vi "Assign two values from string to axes.vi"(2 "Queried axes":string[](array[string]), 4 "Input String":string, 5 "error in":errorcluster) -> (14 "Values 1":dbl[](array[numeric]) format="%.6f", 15 "Strings 1":string[](array[string]), 16 "Values 2":dbl[](array[numeric]) format="%.6f", 17 "Strings 2":string[](array[string]), 18 "Queried axes out":string[](array[string]), 19 "error out":errorcluster)   [LabVIEW 2020]
doc: "This VI assigns two values and/or strings from input string to queried axes."
panel:
  # "This vi assigns two values and/or strings from input string to queried axes."
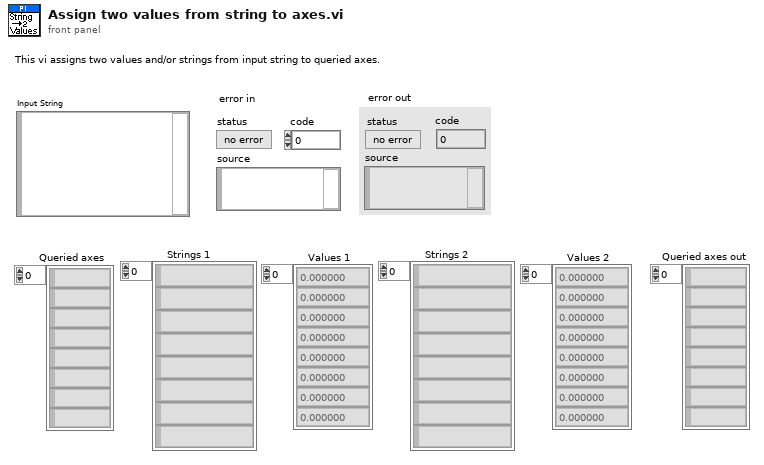
[diagram p1: front panel]
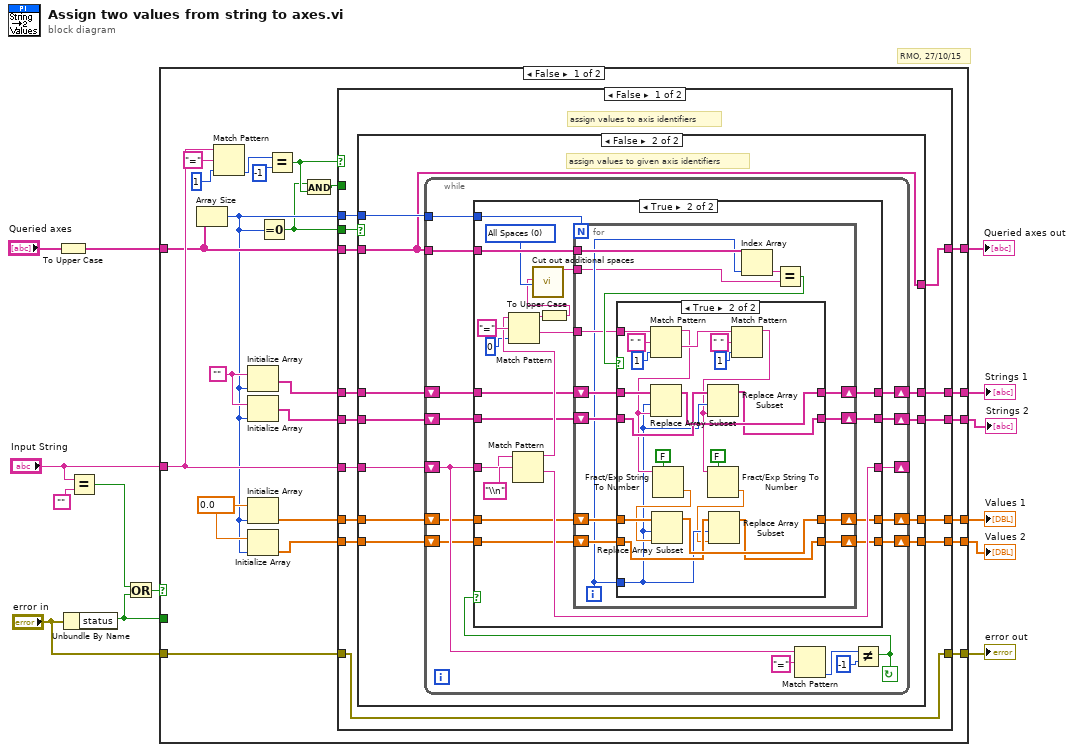
[diagram p0: block diagram]
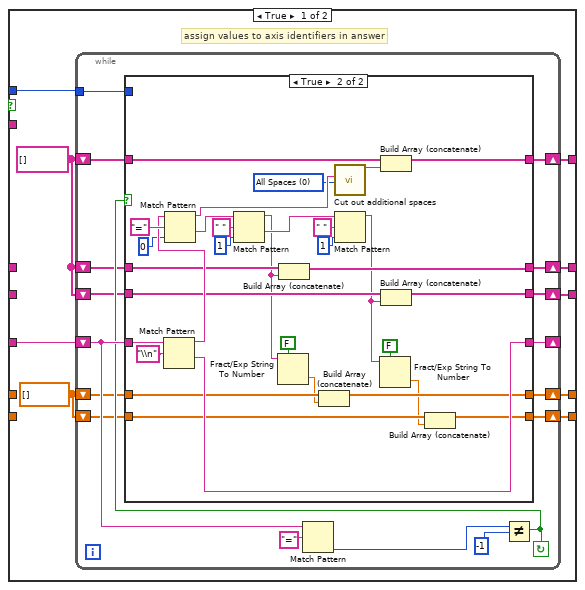
[diagram p2: hidden frame]
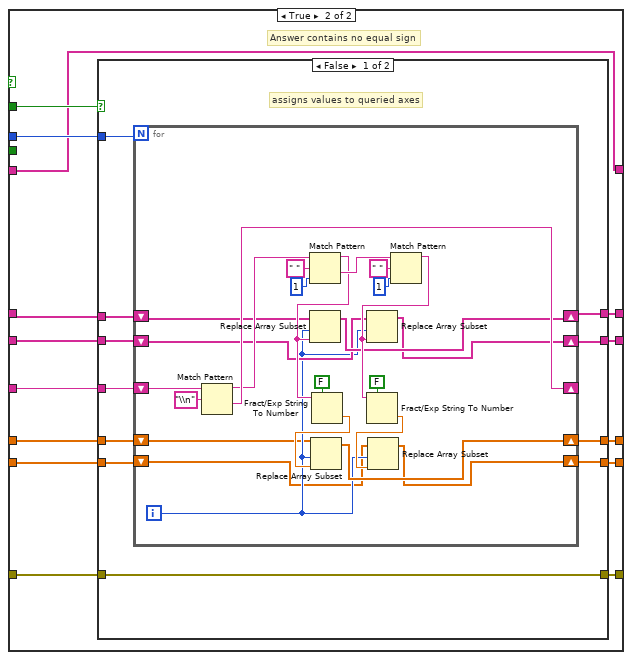
[diagram p6: hidden frame]
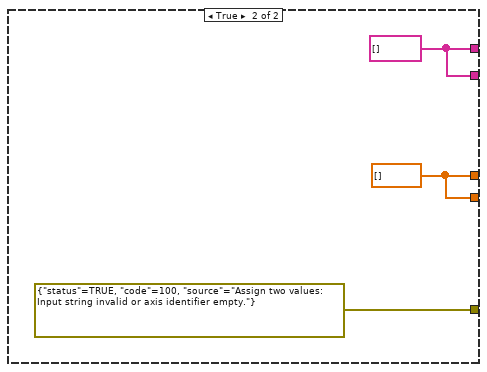
[diagram p7: hidden frame]
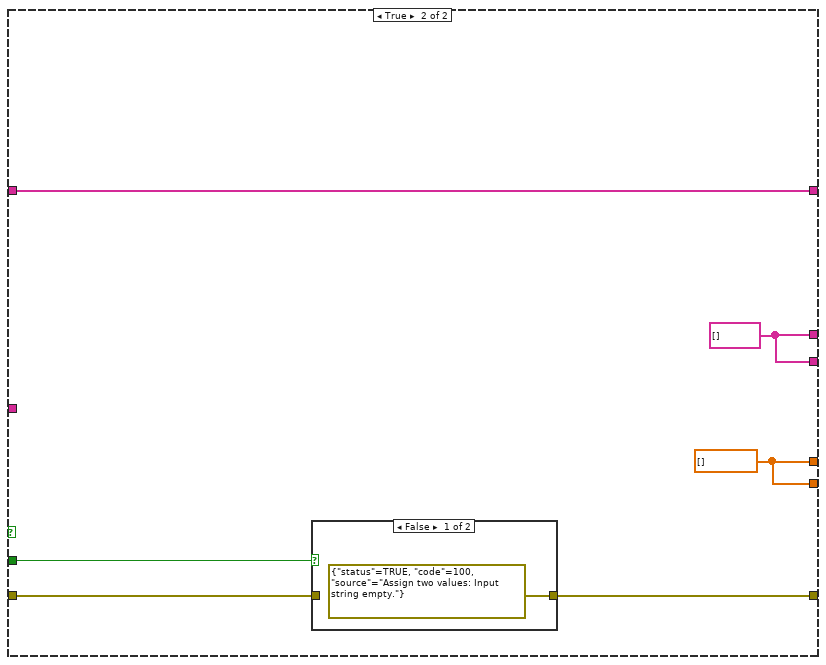
[diagram p8: hidden frame]
diagram:
  # "RMO, 27/10/15"
  n1 = To Upper Case(1:"Queried axes") -> (0:w5:string[])
  n2 = Unbundle By Name("error in") -> ("status"=w7:bool)
  n3 = Equal?(x="Input String", y="") -> (x = y?=w4:bool)
  n4 = Or(x=w4, y=w7) -> (x .or. y?=w9:bool)
  n5 = case shown="False" w9 {
    tunnel: "Input String" -> [w37 _]
    tunnel: [w36 w260] -> w14
    tunnel: w5 -> [w27 w259]
    tunnel: [w25 w263] -> w11
    tunnel: "error in" -> [w24 w264]
    tunnel: [w35 w261] -> w8
    tunnel: w7 -> [_ w262]
    tunnel: [w19 w261] -> w3
    tunnel: [w18 w260] -> w2
    tunnel: [w17 w259] -> w1
    frame False {
      w21 = 0.0 ("Element Data")
      w23 = ""
      n6 = Array Size(array=w27) -> (size(s)=w16:i32)
      n7 = Match Pattern(string=w37, regular expression="=", offset (0)=1) -> (offset past match=w32:i32)  [unwired: 3 out]
      n8 = Initialize Array(w23, w16) -> (w30:string[])
      n9 = Initialize Array(w23, w16) -> (w22:string[])
      n10 = Initialize Array(w21, w16) -> (w31:dbl[])
      n11 = Initialize Array(w21, w16) -> (w20:dbl[])
      n12 = Equal To 0?(x=w16) -> (x = 0?=w15:bool)
      n13 = Equal?(x=w32, y=-1) -> (x = y?=w28:bool)
      n14 = And(x=w15, y=w28) -> (x .and. y?=w26:bool)
      n15 = case shown="False" w28 {
        tunnel: [w50 w220] -> w36
        tunnel: w37 -> [w51 w219]
        tunnel: w27 -> [w40 w209]
        tunnel: w31 -> [w48 w218]
        tunnel: w16 -> [w49 w217]
        tunnel: w30 -> [w47 w216]
        tunnel: [w46 w215] -> w35
        tunnel: w26 -> [_ w214]
        tunnel: [w45 w213] -> w25
        tunnel: w24 -> [w45 w212]
        tunnel: [w44 w211] -> w19
        tunnel: w22 -> [w43 w208]
        tunnel: w20 -> [w42 w207]
        tunnel: [w41 w210] -> w18
        tunnel: [w38 w209] -> w17
        tunnel: w15 -> [w39 _]
        frame False {
          # "assign values to axis identifiers"
          n16 = case shown="False" w39 {
            tunnel: w51 -> [w60 w125]
            tunnel: [w59 w124] -> w50
            tunnel: w49 -> [w58 w123]
            tunnel: w48 -> [_ w122]
            tunnel: w47 -> [_ w121]
            tunnel: [w57 w120] -> w46
            tunnel: [w56 w119] -> w44
            tunnel: w43 -> [_ w118]
            tunnel: w42 -> [_ w117]
            tunnel: [w55 w116] -> w41
            tunnel: w40 -> [_ w115]
            tunnel: [w54 w115] -> w38
            frame True {
              w52 = dbl[] []
              w53 = string[] []
              # "assign values to axis identifiers in answer"
              n17 = while {
                shift-left: w53 -> [w67]
                shift-right: [w68] -> w57
                tunnel: w58 -> [w69]
                shift-left: w52 -> [w71]
                shift-right: [w70] -> w59
                shift-left: w60 -> [w74]
                shift-right: [w73] -> _
                shift-right: [w66] -> w56
                shift-left: w53 -> [w65]
                shift-right: [w64] -> w55
                shift-left: w52 -> [w63]
                shift-right: [w62] -> w54
                shift-left: w53 -> [w61]
                stop <- w72 continue-if-true
                n18 = Match Pattern(string=w74, regular expression="=") -> (offset past match=w75:i32)  [unwired: 4 out]
                n19 = Not Equal?(x=w75, y=-1) -> (x != y?=w72:bool)
                n20 = case shown="True" w72 {
                  tunnel: w74 -> [w83 w113]
                  tunnel: [w83 w112] -> w73
                  tunnel: [w82 w88] -> w70
                  tunnel: w71 -> [w82 w89]
                  tunnel: w69 -> [_ _]
                  tunnel: [w81 w94] -> w68
                  tunnel: w67 -> [w81 w95]
                  tunnel: [w80 w92] -> w66
                  tunnel: w65 -> [w80 w93]
                  tunnel: [w79 w84] -> w64
                  tunnel: w63 -> [w79 w86]
                  tunnel: [w78 w106] -> w62
                  tunnel: w61 -> [w78 w96]
                  frame False {
                    # "line contains no equal sign"
                  }
                  frame True {
                    w98 = u16 0 items=["All Spaces", "Only if 1st char.", "Only if last char.", "Only if near \"=\"", "Only if 1st or last char.", "Only multiple"] ("Mode")
                    n21 = Match Pattern(string=w113, regular expression="\\n") -> (before substring=w110:string, after substring=w112:string)  [unwired: 3 out]
                    n22 = Match Pattern(string=w110, regular expression="=", offset (0)=0) -> (before substring=w107:string, after substring=w109:string)  [unwired: 2 out]
                    n23 = Match Pattern(string=w109, regular expression=" ", offset (0)=1) -> (before substring=w91:string, after substring=w101:string)  [unwired: 2 out]
                    n24 = Fract/Exp String To Number(use system decimal point (T)=FALSE, string=w91) -> (number=w87:dbl)  [unwired: 3 out]
                    n25 = Build Array (concatenate)(w95, w91) -> (w94:string[])
                    n26 = Build Array (concatenate)(w89, w87) -> (w88:dbl[])
                    n27 = call "Cut out additional spaces.vi"("String"=w107, "Mode"=w98) -> ("String out"=w97:string)  [unwired: 17 out]
                    n28 = Match Pattern(string=w101, regular expression=" ", offset (0)=1) -> (before substring=w90:string)  [unwired: 3 out]
                    n29 = Fract/Exp String To Number(use system decimal point (T)=FALSE, string=w90) -> (number=w85:dbl)  [unwired: 3 out]
                    n30 = Build Array (concatenate)(w96, w97) -> (w106:string[])
                    n31 = Build Array (concatenate)(w93, w90) -> (w92:string[])
                    n32 = Build Array (concatenate)(w86, w85) -> (w84:dbl[])
                  }
                }
              }
            }
            frame False {
              # "assign values to given axis identifiers"
              n33 = while {
                shift-left: w121 -> [w130]
                shift-right: [w131] -> w120
                tunnel: w123 -> [w132]
                tunnel: w115 -> [w133]
                shift-left: w122 -> [w135]
                shift-right: [w134] -> w124
                shift-left: w125 -> [w138]
                shift-right: [w137] -> _
                shift-right: [w129] -> w119
                shift-left: w118 -> [w128]
                shift-right: [w127] -> w116
                shift-left: w117 -> [w126]
                stop <- w136 continue-if-true
                n34 = Match Pattern(string=w138, regular expression="=") -> (offset past match=w139:i32)  [unwired: 4 out]
                n35 = Not Equal?(x=w139, y=-1) -> (x != y?=w136:bool)
                n36 = case shown="True" w136 {
                  tunnel: w138 -> [w146 w166]
                  tunnel: [w146 w165] -> w137
                  tunnel: [w145 w163] -> w134
                  tunnel: w135 -> [w145 w164]
                  tunnel: w133 -> [_ w160]
                  tunnel: w132 -> [_ w158]
                  tunnel: [w144 w156] -> w131
                  tunnel: w130 -> [w144 w155]
                  tunnel: [w143 w153] -> w129
                  tunnel: w128 -> [w143 w152]
                  tunnel: [w142 w151] -> w127
                  tunnel: w126 -> [w142 w150]
                  frame False {
                  }
                  frame True {
                    w149 = u16 0 items=["All Spaces", "Only if 1st char.", "Only if last char.", "Only if near \"=\"", "Only if 1st or last char.", "Only multiple"] ("Mode")
                    n37 = Match Pattern(string=w166, regular expression="\\n") -> (before substring=w161:string, after substring=w165:string)  [unwired: 3 out]
                    n38 = Match Pattern(string=w161, regular expression="=", offset (0)=0) -> (before substring=w159:string, after substring=w157:string)  [unwired: 2 out]
                    n39 = To Upper Case(1:w159) -> (0:w148:string)
                    n40 = call "Cut out additional spaces.vi"("String"=w148, "Mode"=w149) -> ("String out"=w147:string)  [unwired: 17 out]
                    n41 = for {
                      N: w158 -> [_]
                      shift-right: [w180] -> w163
                      shift-left: w164 -> [w181]
                      tunnel: w160 -> [w179]
                      tunnel: w147 -> [w168]
                      shift-right: [w175] -> w156
                      shift-left: w155 -> [w176]
                      tunnel: w157 -> [w172]
                      shift-right: [w174] -> w153
                      shift-left: w152 -> [w173]
                      shift-right: [w170] -> w151
                      shift-left: w150 -> [w171]
                      i -> [w169]
                      n42 = Index Array(array=w179, index=w169) -> (element=w178:string)
                      n43 = Equal?(x=w178, y=w168) -> (x = y?=w177:bool)
                      n44 = case shown="True" w177 {
                        tunnel: w169 -> [_ w190]
                        tunnel: w181 -> [w185 w206]
                        tunnel: [w185 w205] -> w180
                        tunnel: w176 -> [w184 w204]
                        tunnel: [w184 w203] -> w175
                        tunnel: [w183 w202] -> w174
                        tunnel: w173 -> [w183 w201]
                        tunnel: w172 -> [_ w200]
                        tunnel: w171 -> [w182 w191]
                        tunnel: [w182 w189] -> w170
                        frame False {
                        }
                        frame True {
                          n45 = Match Pattern(string=w200, regular expression=" ", offset (0)=1) -> (before substring=w193:string, after substring=w195:string)  [unwired: 2 out]
                          n46 = Replace Array Subset(array=w204, new element=w193, index=w190) -> (w203:string[])
                          n47 = Fract/Exp String To Number(use system decimal point (T)=FALSE, string=w193) -> (number=w192:dbl)  [unwired: 3 out]
                          n48 = Replace Array Subset(array=w206, new element=w192, index=w190) -> (w205:dbl[])
                          n49 = Match Pattern(string=w195, regular expression=" ", offset (0)=1) -> (before substring=w187:string)  [unwired: 3 out]
                          n50 = Replace Array Subset(array=w201, new element=w187, index=w190) -> (w202:string[])
                          n51 = Fract/Exp String To Number(use system decimal point (T)=FALSE, string=w187) -> (number=w186:dbl)  [unwired: 3 out]
                          n52 = Replace Array Subset(array=w191, new element=w186, index=w190) -> (w189:dbl[])
                        }
                      }
                    }
                  }
                }
              }
            }
          }
        }
        frame True {
          # "Answer contains no equal sign"
          n53 = case shown="False" w214 {
            tunnel: [w231 w256] -> w220
            tunnel: w219 -> [w230 _]
            tunnel: w218 -> [w229 _]
            tunnel: w217 -> [w228 _]
            tunnel: w216 -> [w225 _]
            tunnel: [w227 w257] -> w215
            tunnel: [w226 errorcluster {"status"=TRUE, "code"=100, "source"="Assign two values: Input string invalid or axis identifier empty."} ("error out")] -> w213
            tunnel: w212 -> [w226 _]
            tunnel: [w221 w257] -> w211
            tunnel: [w222 w256] -> w210
            tunnel: w208 -> [w224 _]
            tunnel: w207 -> [w223 _]
            frame False {
              # "assigns values to queried axes"
              n54 = for {
                N: w228 -> [_]
                shift-right: [w237] -> w231
                shift-left: w229 -> [w233]
                shift-right: [w254] -> _
                shift-left: w230 -> [w255]
                shift-right: [w239] -> w227
                shift-left: w225 -> [w240]
                shift-right: [w238] -> w221
                shift-left: w224 -> [w235]
                shift-right: [w236] -> w222
                shift-left: w223 -> [w232]
                i -> [w234]
                n55 = Match Pattern(string=w255, regular expression="\\n") -> (before substring=w241:string, after substring=w254:string)  [unwired: 3 out]
                n56 = Match Pattern(string=w241, regular expression=" ", offset (0)=1) -> (before substring=w246:string, after substring=w248:string)  [unwired: 2 out]
                n57 = Replace Array Subset(array=w240, new element=w246, index=w234) -> (w239:string[])
                n58 = Fract/Exp String To Number(use system decimal point (T)=FALSE, string=w246) -> (number=w245:dbl)  [unwired: 3 out]
                n59 = Replace Array Subset(array=w233, new element=w245, index=w234) -> (w237:dbl[])
                n60 = Match Pattern(string=w248, regular expression=" ", offset (0)=1) -> (before substring=w243:string)  [unwired: 3 out]
                n61 = Replace Array Subset(array=w235, new element=w243, index=w234) -> (w238:string[])
                n62 = Fract/Exp String To Number(use system decimal point (T)=FALSE, string=w243) -> (number=w242:dbl)  [unwired: 3 out]
                n63 = Replace Array Subset(array=w232, new element=w242, index=w234) -> (w236:dbl[])
              }
            }
            frame True {
              w256 = dbl[] []
              w257 = string[] []
            }
          }
        }
      }
    }
    frame True {
      w261 = string[] []
      w260 = dbl[] [] ("Step Size")
      # "Error"
      n64 = case shown="False" w262 {
        tunnel: w264 -> [_ w266]
        tunnel: [errorcluster {"status"=TRUE, "code"=100, "source"="Assign two values: Input string empty."} ("error out") w266] -> w263
        frame False {
        }
        frame True {
        }
      }
    }
  }
  "Values 1" <- w14
  "error out" <- w11
  "Strings 1" <- w8
  "Strings 2" <- w3
  "Values 2" <- w2
  "Queried axes out" <- w1
